vi "备份参数.vi"() -> (0 "仪器公式":T1(array[cluster]), 1 "量程参数":T2(array[cluster]), 2 "试剂容量参数":T3, 3 "外设参数":cluster{"外设配置":T4, "error out":errorcluster} {"外设配置"."阀方向" items=["顺时针", "逆时针", "就近"]; "外设配置"."总氮x公式0" items=["0", "1"]; "外设配置"."光谱仪类型" items=["1型", "2型", "3型", "2型氙灯联控"]; "外设配置"."泵阀量" items=["9通"=9, "10通"=10, "12通"=12]; "外设配置"."泵类型" items=["1型", "2型", "sy04型+旋转阀"]}, 5 "备份结果":string)   [LabVIEW 2016, in "斯坦道总磷.lvlib"]
uses:
  <vilib>/NI/Progress Bar/Progress Bar.lvlib
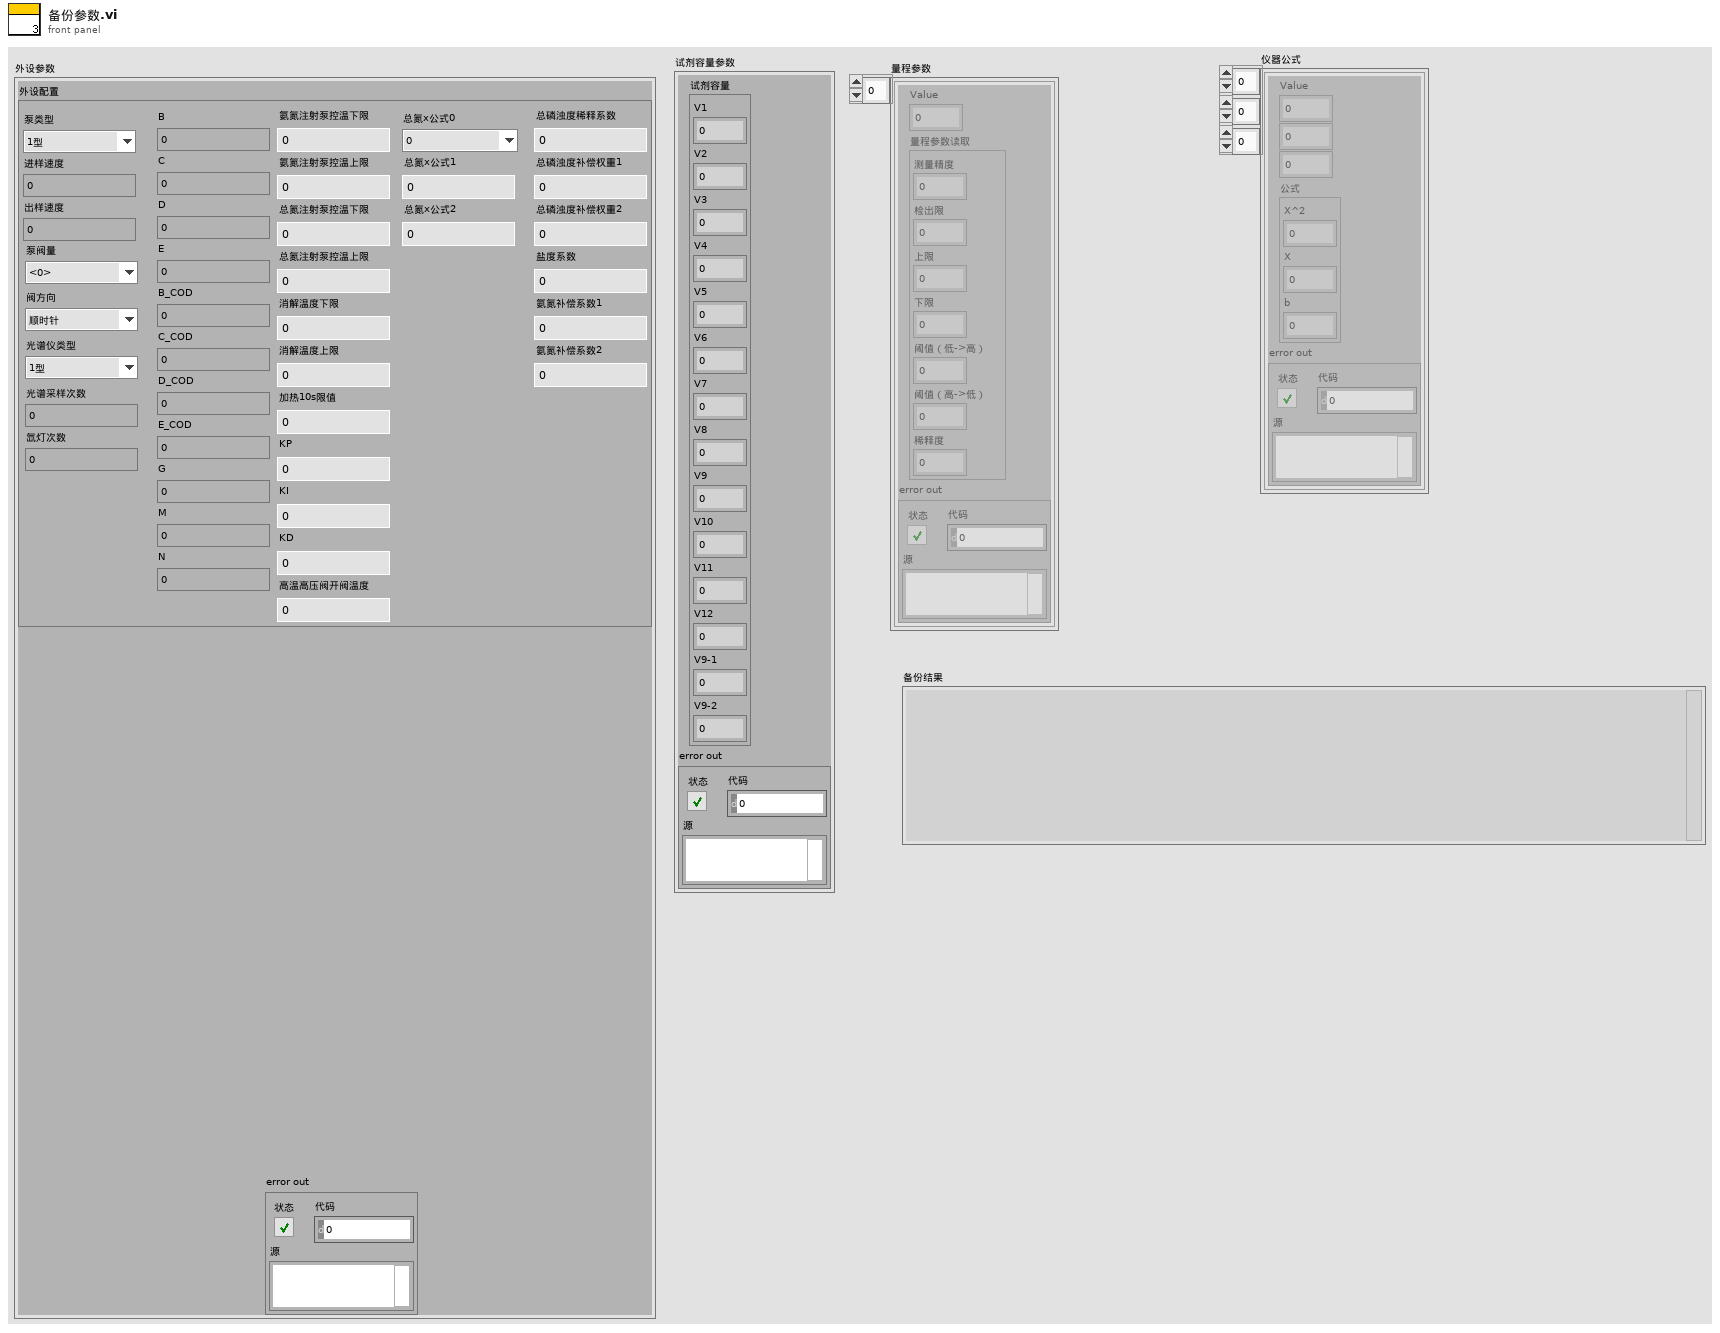
[diagram p1: front panel]
types:
  T1 = cluster{"Value":u16, i32, i32, "公式":cluster{"X^2":dbl, "X":dbl, "b":dbl}, "error out":errorcluster}[][][]
  T2 = cluster{"Value":u16, "量程参数读取":cluster{"测量精度":u16, "检出限":dbl, "上限":dbl, "下限":dbl, "阈值（低->高）":dbl, "阈值（高->低）":dbl, "稀释度":dbl}, "error out":errorcluster}[]
  T3 = cluster{"试剂容量":cluster{"V1":sgl, "V2":sgl, "V3":sgl, "V4":sgl, "V5":sgl, "V6":sgl, "V7":sgl, "V8":sgl, "V9":sgl, "V10":sgl, "V11":sgl, "V12":sgl, "V9-1":sgl, "V9-2":sgl}, "error out":errorcluster}
  T4 = typedef "斯坦道总磷.lvlib/V3 A版外设参数.ctl" = cluster{"泵类型":u8, "进样速度":u32, "出样速度":u32, "泵阀量":u8, "阀方向":u8, "光谱仪类型":u8, "光谱采样次数":u8, "氙灯次数":u8, "B":u16, "C":u16, "D":u16, "E":u16, "B_COD":u16, "C_COD":u16, "D_COD":u16, "E_COD":u16, "G":u16, "M":u16, "N":u16, "氨氮注射泵控温下限":sgl, "氨氮注射泵控温上限":sgl, "总氮注射泵控温下限":sgl, "总氮注射泵控温上限":sgl, "消解温度下限":sgl, "消解温度上限":sgl, "加热10s限值":sgl, "KP":sgl, "KI":sgl, "KD":sgl, "高温高压阀开阀温度":sgl, "总氮x公式0":u8, "总氮x公式1":sgl, "总氮x公式2":sgl, "总磷浊度稀释系数":sgl, "总磷浊度补偿权重1":sgl, "总磷浊度补偿权重2":sgl, "盐度系数":sgl, "氨氮补偿系数1":sgl, "氨氮补偿系数2":sgl}
  T5 = enum16{"备份外设参数", "备份试剂容量参数", "备份量程参数", "备份仪器公式", "结束"}
  T6 = cluster{"V1":sgl, "V2":sgl, "V3":sgl, "V4":sgl, "V5":sgl, "V6":sgl, "V7":sgl, "V8":sgl, "V9":sgl, "V10":sgl, "V11":sgl, "V12":sgl, "V9-1":sgl, "V9-2":sgl}
  T7 = cluster{"测量精度":u16, "检出限":dbl, "上限":dbl, "下限":dbl, "阈值（低->高）":dbl, "阈值（高->低）":dbl, "稀释度":dbl}
  T8 = cluster{"Value":u16, "量程参数读取":cluster{"测量精度":u16, "检出限":dbl, "上限":dbl, "下限":dbl, "阈值（低->高）":dbl, "阈值（高->低）":dbl, "稀释度":dbl}, "error out":errorcluster}
  T9 = cluster{"Value":u16, i32, i32, "公式":cluster{"X^2":dbl, "X":dbl, "b":dbl}, "error out":errorcluster}
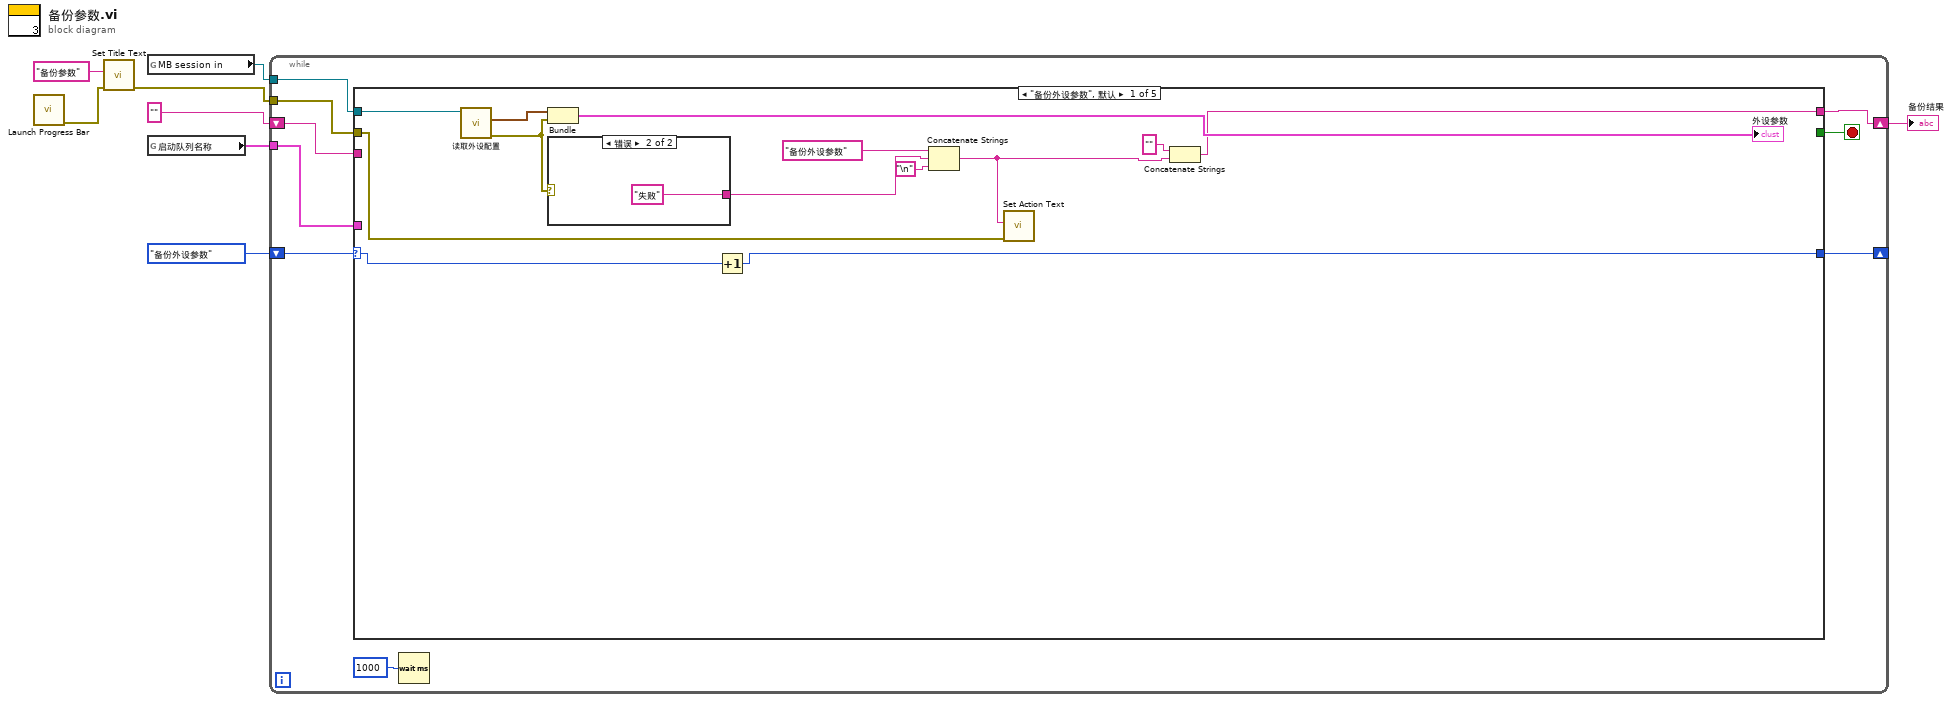
[diagram p0: block diagram]
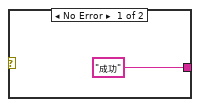
[diagram p2: hidden frame]
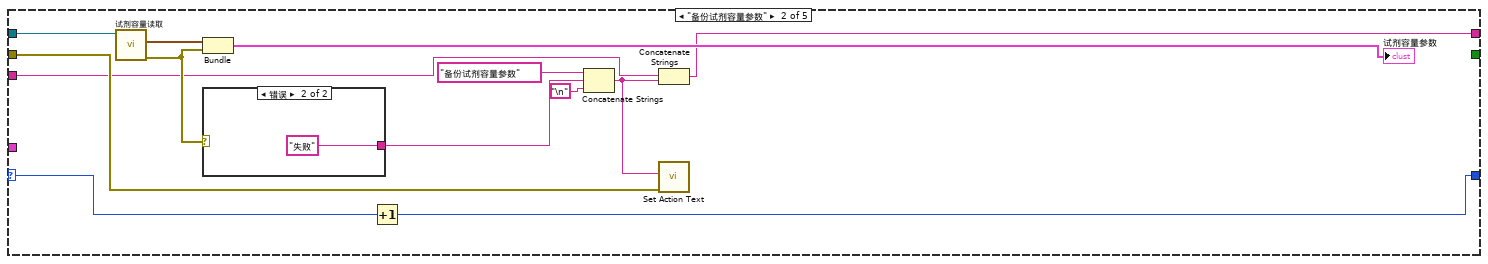
[diagram p3: hidden frame]
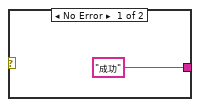
[diagram p4: hidden frame]
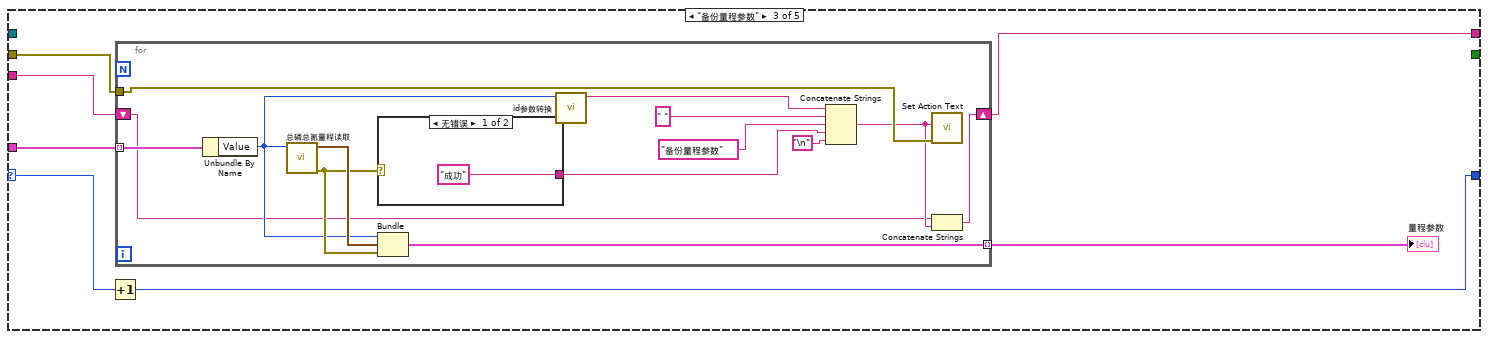
[diagram p5: hidden frame]
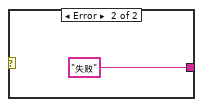
[diagram p6: hidden frame]
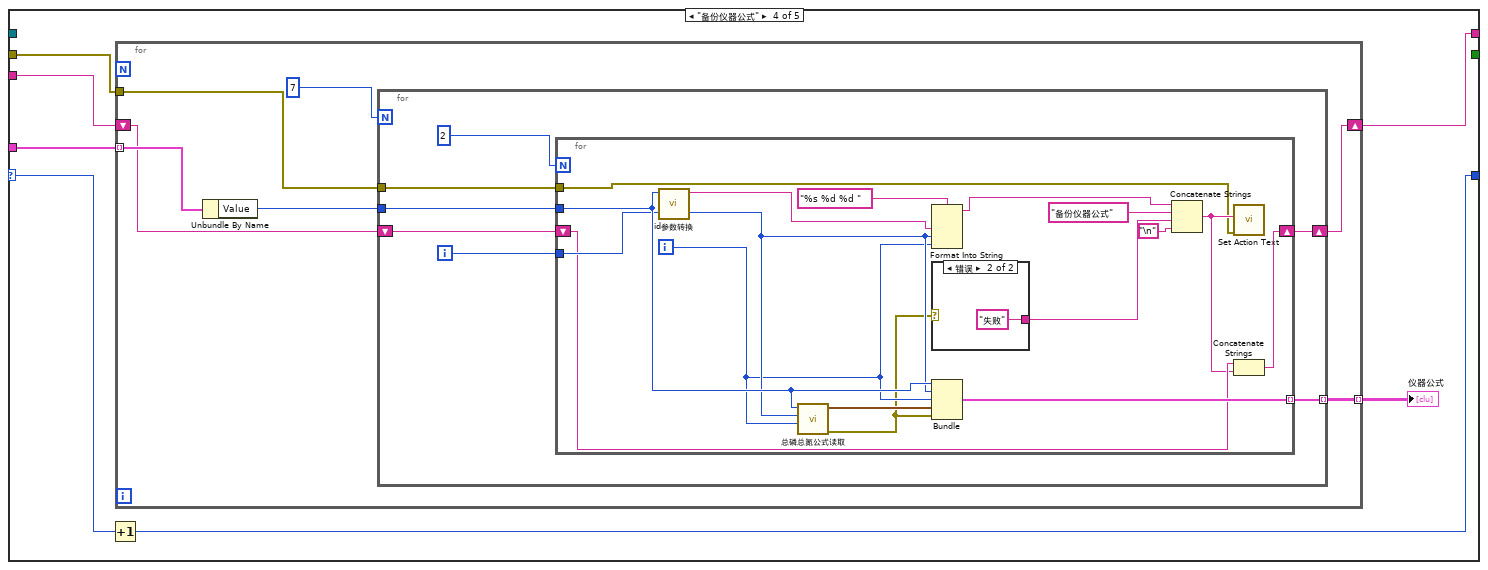
[diagram p7: hidden frame]
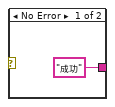
[diagram p8: hidden frame]
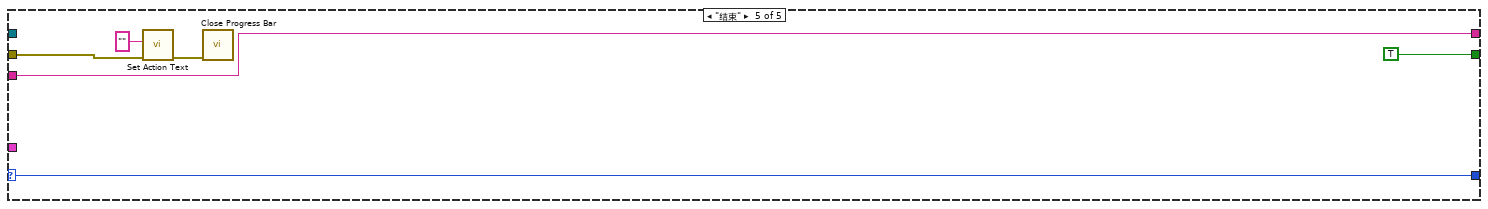
[diagram p9: hidden frame]
diagram:
  n1 = call <vilib>:"Launch Progress Bar.vi"() -> ("error out"=w3:errorcluster)  [unwired: 10 in, 1 out]
  n2 = call <vilib>:"Set Title Text.vi"("error in (no error)"=w3, "Installer Title"="备份参数") -> ("error out"=w2:errorcluster)  [unwired: 9 in]
  n3 = global read "VAR总磷总氮全局变量.vi" "MB session in"() -> (w7:refnum<class "MB_Master.lvclass">)
  n4 = global read "model config var.vi" "启动队列名称"() -> (w5:cluster{"String":string, "Value":u16}[])
  n5 = while {
    shift-right: [w13] -> _
    shift-left: T5."备份外设参数" ("枚举") -> [w16]
    tunnel: w7 -> [w17]
    shift-right: [w14] -> w4
    shift-left: "" -> [w15]
    tunnel: w5 -> [w12]
    tunnel: w2 -> [w10]
    stop <- w11 stop-if-true
    n6 = case shown="\"备份外设参数\", 默认" w16 {
      selector: w16 -> [w24 w39 w51 w74 w115]
      tunnel: w17 -> [w30 w45 _ _ _]
      tunnel: w15 -> [_ w35 w53 w76 w114]
      tunnel: [w20 w33 w52 w75 w114] -> w14
      tunnel: [w23 w38 w50 w73 w115] -> w13
      tunnel: w12 -> [_ _ w54 w77 _]
      tunnel: [_ _ _ _ TRUE] -> w11
      tunnel: w10 -> [w18 w36 w48 w71 w112]
      frame "备份外设参数", Default {
        n7 = call "读取外设配置.vi"("MB session in"=w30) -> ("error out"=w28:errorcluster, "外设配置"=w29:T4)  [unwired: 8 in, 1 out]
        n8 = Bundle("外设配置"=w29, "error out"=w28) -> (→"外设参数":cluster{"外设配置":T4, "error out":errorcluster})  [unwired: 1 in]
        n9 = case shown="错误" w28 {
          tunnel: ["成功" "失败"] -> w27
          frame No Error {
          }
          frame Error {
          }
        }
        n10 = Increment(x=w24) -> (x+1=w23:T5)
        n11 = Concatenate Strings("备份外设参数" ("字符串"), w27, "\n") -> (w21:string)
        n12 = call <vilib>:"Set Action Text.vi"("error in (no error)"=w18, "Action Text"=w21) -> ()  [unwired: 9 in, 1 out]
        n13 = Concatenate Strings("" ("字符串"), w21) -> (w20:string)
      }
      frame "备份试剂容量参数" {
        n14 = call "试剂容量读取.vi"("MB session in"=w45) -> ("error out"=w40:errorcluster, "试剂容量"=w44:T6)  [unwired: 8 in, 1 out]
        n15 = Bundle("试剂容量"=w44, "error out"=w40) -> (→"试剂容量参数":T3)  [unwired: 1 in]
        n16 = case shown="错误" w40 {
          tunnel: ["成功" "失败"] -> w43
          frame No Error {
          }
          frame Error {
          }
        }
        n17 = Increment(x=w39) -> (x+1=w38:T5)
        n18 = Concatenate Strings("备份试剂容量参数" ("字符串"), w43, "\n") -> (w34:string)
        n19 = Concatenate Strings(w35, w34) -> (w33:string)
        n20 = call <vilib>:"Set Action Text.vi"("error in (no error)"=w36, "Action Text"=w34) -> ()  [unwired: 9 in, 1 out]
      }
      frame "备份量程参数" {
        n21 = Increment(x=w51) -> (x+1=w50:T5)
        n22 = for {
          tunnel: w54 -> [w68] mode=indexing
          tunnel: [w66] -> w49 mode=indexing
          shift-right: [w55] -> w52
          shift-left: w53 -> [w56]
          tunnel: w48 -> [w58]
          n23 = Unbundle By Name(w68) -> ("Value"=w62:u16)
          n24 = call "总磷总氮量程读取.vi"("测量参数"=w62) -> ("error out"=w63:errorcluster, "量程参数读取"=w67:T7)  [unwired: 9 in]
          n25 = case shown="无错误" w63 {
            tunnel: ["成功" "失败"] -> w65
            frame No Error {
            }
            frame Error {
            }
          }
          n26 = Bundle("Value"=w62, "量程参数读取"=w67, "error out"=w63) -> (w66:T8)  [unwired: 1 in]
          n27 = call "id参数转换.vi"("id"=w62) -> ("table输出"=w61:string)  [unwired: 9 in, 1 out]
          n28 = Concatenate Strings(w61, " " ("字符串"), "备份量程参数" ("字符串"), w65, "\n") -> (w57:string)
          n29 = call <vilib>:"Set Action Text.vi"("error in (no error)"=w58, "Action Text"=w57) -> ()  [unwired: 9 in, 1 out]
          n30 = Concatenate Strings(w56, w57) -> (w55:string)
        }
        "量程参数" <- w49
      }
      frame "备份仪器公式" {
        n31 = Increment(x=w74) -> (x+1=w73:T5)
        n32 = for {
          tunnel: w77 -> [w84] mode=indexing
          tunnel: [w81] -> w72 mode=indexing
          shift-right: [w79] -> w75
          shift-left: w76 -> [w80]
          tunnel: w71 -> [w78]
          n33 = Unbundle By Name(w84) -> ("Value"=w82:u16)
          n34 = for {
            N: 7 -> [_]
            tunnel: w82 -> [w91]
            tunnel: [w88] -> w81 mode=indexing
            shift-right: [w87] -> w79
            shift-left: w80 -> [w86]
            tunnel: w78 -> [w85]
            i -> [w90]
            n35 = for {
              N: 2 -> [_]
              tunnel: w91 -> [w103]
              tunnel: w90 -> [w100]
              tunnel: [w106] -> w88 mode=indexing
              shift-right: [w92] -> w87
              shift-left: w86 -> [w95]
              tunnel: w85 -> [w93]
              i -> [w99]
              n36 = call "id参数转换.vi"("id"=w103) -> ("table输出"=w101:string)  [unwired: 9 in, 1 out]
              n37 = call "总磷总氮公式读取.vi"("量程"=w99, "测量模式"=w100, "测量参数"=w103) -> ("error out"=w97:errorcluster, "公式"=w107:cluster{"X^2":dbl, "X":dbl, "b":dbl})  [unwired: 7 in]
              n38 = Format Into String(format string="%s %d %d " ("格式字符串"), w101, w100, w99) -> (resulting string=w98:string)  [unwired: 2 in, 1 out]
              n39 = case shown="错误" w97 {
                tunnel: ["成功" "失败"] -> w105
                frame No Error {
                }
                frame Error {
                }
              }
              n40 = Bundle("Value"=w103, w100, w99, "公式"=w107, "error out"=w97) -> (w106:T9)  [unwired: 1 in]
              n41 = Concatenate Strings(w98, "备份仪器公式" ("字符串"), w105, "\n") -> (w94:string)
              n42 = call <vilib>:"Set Action Text.vi"("error in (no error)"=w93, "Action Text"=w94) -> ()  [unwired: 9 in, 1 out]
              n43 = Concatenate Strings(w95, w94) -> (w92:string)
            }
          }
        }
        "仪器公式" <- w72
      }
      frame "结束" {
        n44 = call <vilib>:"Set Action Text.vi"("error in (no error)"=w112, "Action Text"="") -> ("error out"=w110:errorcluster)  [unwired: 9 in]
        n45 = call <vilib>:"Close Progress Bar.vi"("error in (no error)"=w110) -> ()  [unwired: 9 in, 2 out]
      }
    }
    n46 = Wait (ms)(milliseconds to wait=u32 1000 ("等待时间（毫秒）")) -> ()  [unwired: 1 out]
  }
  "备份结果" <- w4
